vi "DiscArchiver.unregister from event builder.vi"(0 "i ref in":refnum<vi>, 3 "ms timeout (10000)":i32=10000, 5 "error in (no error)":errorcluster) -> (14 "i ref out":refnum<vi>, 17 "timed out":bool, 19 "error out":errorcluster)   [LabVIEW 2014, in "DiscArchiver.lvlib"]
doc: "Unregisters the DiscArchiver from an EventBuilder object."
uses:
  DiscArchiver.lvlib
  CSCore/CAEObj/CAEObj.lvlib
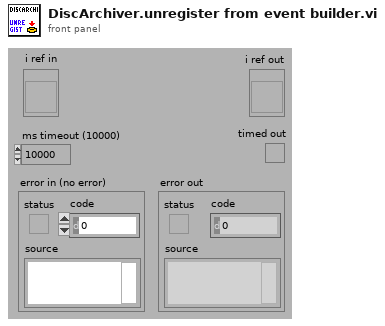
[diagram p1: front panel]
types:
  T1 = typedef "DiscArchiver.lvlib/DiscArchiver.i attribute.ctl" = cluster{"file prefix":string, "actual file":string, "nOfEvents":i32, "file":refnum<file>, "eventBuilder":string, "disc size alarm":bool, "dataDescription":string, "dataDescriptionURL":string, "eventDataURL":string, "headerID":dbl, "completeData":bool, "nOfEventsID":i32, "dataFileID":i32}
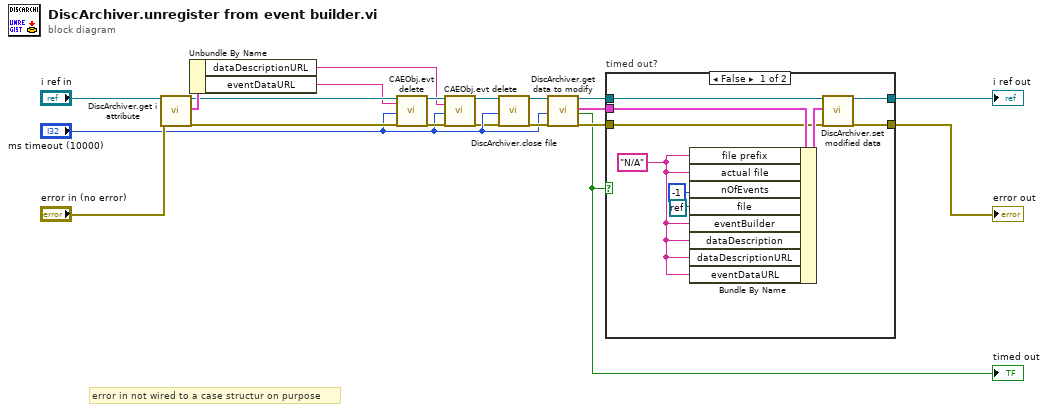
[diagram p0: block diagram]
diagram:
  # "error in not wired to a case structur on purpose"
  n1 = call "DiscArchiver.get i attribute.vi"("i ref in"="i ref in", "error in (no error)"="error in (no error)") -> ("i ref out"=w10:refnum<vi>, "i attribute"=w11:T1, "error out"=w9:errorcluster)  [unwired: 15 in]
  n2 = Unbundle By Name(w11) -> ("dataDescriptionURL"=w5:string, "eventDataURL"=w8:string)
  n3 = call "CAEObj.evt delete.vi"("i ref in"=w10, "URL"=w8, "ms timeout (10000)"="ms timeout (10000)", "error in (no error)"=w9) -> ("i ref out"=w6:refnum<vi>, "error out"=w7:errorcluster)  [unwired: 12 in, 2 out]
  n4 = call "CAEObj.evt delete.vi"("i ref in"=w6, "URL"=w5, "ms timeout (10000)"="ms timeout (10000)", "error in (no error)"=w7) -> ("i ref out"=w3:refnum<vi>, "error out"=w1:errorcluster)  [unwired: 12 in, 2 out]
  n5 = call "DiscArchiver.close file.vi"("i ref in"=w3, "ms timeout (10000)"="ms timeout (10000)", "error in (no error)"=w1) -> ("i ref out"=w15:refnum<vi>, "error out"=w14:errorcluster)  [unwired: 14 in, 1 out]
  n6 = call "DiscArchiver.get data to modify.vi"("i ref in"=w15, "ms timeout (10000)"="ms timeout (10000)", "error in (no error)"=w14) -> ("i ref out"=w19:refnum<vi>, "i attribute"=w17:T1, "timed out"=w16:bool, "error out"=w18:errorcluster)  [unwired: 13 in]
  "timed out" <- w16
  n7 = case "timed out?" shown="False" w16 {
    tunnel: [w29 w30] -> w2
    tunnel: [w28 w31] -> w20
    tunnel: w19 -> [w25 w31]
    tunnel: w18 -> [w24 w30]
    tunnel: w17 -> [w26 _]
    frame False {
      w23 = "N/A" ("file prefix")
      n8 = Bundle By Name(cluster=w26, "file prefix"=w23, "actual file"=w23, "nOfEvents"=-1 ("# of items"), "file"=refnum<k0> refnum, "eventBuilder"=w23, "dataDescription"=w23, "dataDescriptionURL"=w23, "eventDataURL"=w23) -> (w27:T1)
      n9 = call "DiscArchiver.set modified data.vi"("i ref in"=w25, "i attribute"=w27, "error in (no error)"=w24) -> ("i ref out"=w28:refnum<vi>, "error out"=w29:errorcluster)  [unwired: 15 in]
    }
    frame True {
    }
  }
  "error out" <- w2
  "i ref out" <- w20
